vi "RT.vi"   [LabVIEW 2016]
uses:
  rt state control.ctl
  commands.ctl
  <vilib>/FPGAPlugInAG/cRIO-9067/niLvFpga_Open_cRIO-9067.vi
  <vilib>/rvi/interface/common/dynamic/niFpgaDynamicAddResources.vi
  <vilib>/Utility/error.llb/Error Cluster From Error Code.vi
  <vilib>/rvi/errors/niLvFpgaAdjustHostInterfaceError.vi
  <vilib>/rvi/interface/nirviOpenFPGA/nirviOpenFPGA.xnode
  FPGA Bitfiles/NSV-events_FPGATarget_test-FPGA_MCVqyRuBWmI.lvbitx
  FPGA.vi
  <vilib>/rvi/interface/nirviReadWriteControl/nirviReadWriteControl.xnode
  NiFpgaLv.dll
  <vilib>/rvi/interface/Simulation/niFpgaSimulationCallBeginRW.vi
  <vilib>/NI_Real-Time Target Support.lvlib
types:
  T1 = typedef "rt state control.ctl" = enum16{"initialize", "wait for update", "process update", "stop"}
  T2 = typedef "commands.ctl" = enum16{"Flash Both", "Stop All Flash", "Flash FPGA", "Stop FPGA Flash", "Flash RT", "Stop RT Flash"}
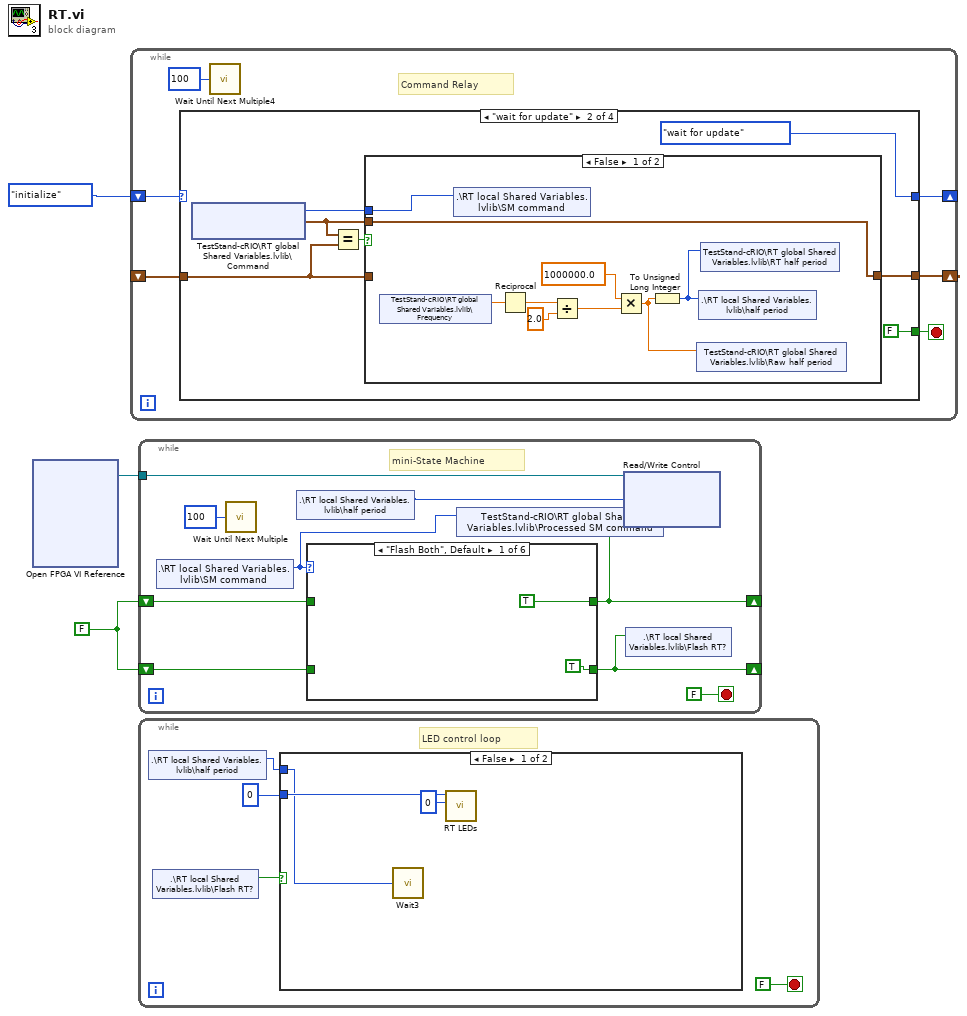
[diagram p0: block diagram]
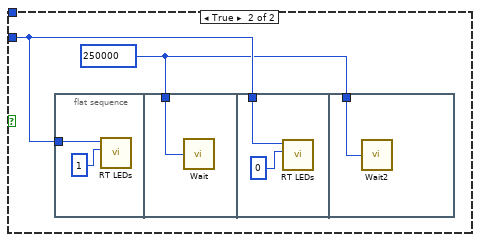
[diagram p2: hidden frame]
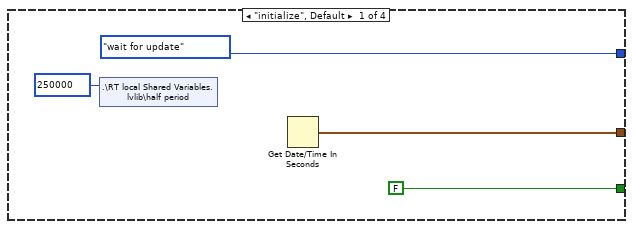
[diagram p3: hidden frame]
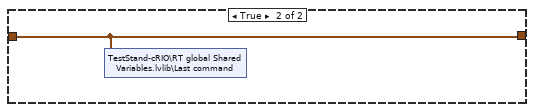
[diagram p4: hidden frame]
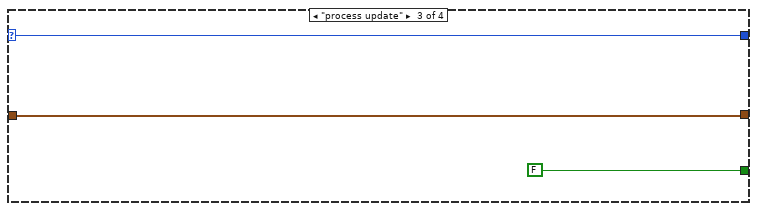
[diagram p5: hidden frame]
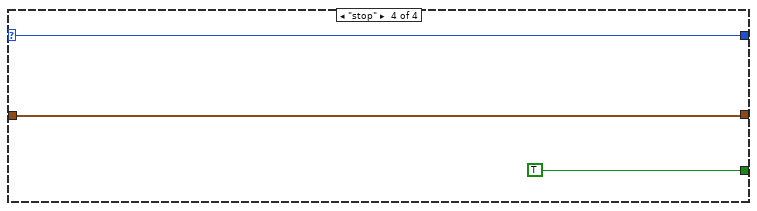
[diagram p6: hidden frame]
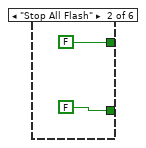
[diagram p7: hidden frame]
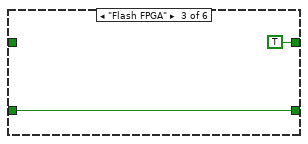
[diagram p8: hidden frame]
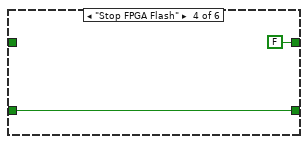
[diagram p9: hidden frame]
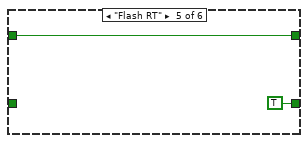
[diagram p10: hidden frame]
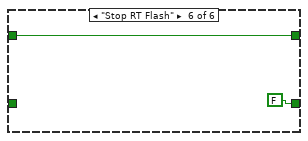
[diagram p11: hidden frame]
diagram:
  w2 = FALSE
  n1 = xnode "Open FPGA VI Reference"() -> ("FPGA VI Reference Out"=w3:refnum<k20>)  [unwired: 2 in, 1 out]
  n2 = while {
    shift-right: [w7] -> _
    shift-left: rt_state_control."initialize" -> [w9]
    shift-right: [w6] -> _
    shift-left: _ -> [w5]
    stop <- w8 stop-if-true
    # "Command Relay"
    n3 = case shown="\"wait for update\"" w9 {
      selector: w9 -> [_ _ w31 w34]
      tunnel: [FALSE FALSE FALSE TRUE] -> w8
      tunnel: [rt_state_control."wait for update" rt_state_control."wait for update" w31 w34] -> w7
      tunnel: [w11 w15 w32 w35] -> w6
      tunnel: w5 -> [_ w16 w32 w35]
      frame "initialize", Default {
        n4 = shared-variable ".\\RT local Shared Variables.lvlib\\half period"(u32 250000 ("half period")) -> ()  [unwired: 1 in, 1 out]
        n5 = Get Date/Time In Seconds() -> (seconds since 1Jan1904=w11:timestamp)
      }
      frame "wait for update" {
        n6 = shared-variable "TestStand-cRIO\\RT global Shared Variables.lvlib\\Command"() -> (w19:T2, w17:timestamp)  [unwired: 1 in, 1 out]
        n7 = Equal?(x=w17, y=w16) -> (x = y?=w18:bool)
        n8 = case shown="False" w18 {
          tunnel: w19 -> [w28 _]
          tunnel: w17 -> [w29 _]
          tunnel: w16 -> [_ w30]
          tunnel: [w29 w30] -> w15
          frame False {
            n9 = shared-variable "TestStand-cRIO\\RT global Shared Variables.lvlib\\Frequency"() -> (w27:dbl)  [unwired: 1 in, 1 out]
            n10 = shared-variable ".\\RT local Shared Variables.lvlib\\SM command"(w28) -> ()  [unwired: 1 in, 1 out]
            n11 = Reciprocal(x=w27) -> (1/x=w26:dbl)
            n12 = Divide(x=w26, y=2.0) -> (x/y=w24:dbl)
            n13 = Multiply(x=1000000.0, y=w24) -> (x*y=w22:dbl)
            n14 = To Unsigned Long Integer(number=w22) -> (unsigned 32bit integer=w21:u32)
            n15 = shared-variable "TestStand-cRIO\\RT global Shared Variables.lvlib\\Raw half period"(w22) -> ()  [unwired: 1 in, 1 out]
            n16 = shared-variable ".\\RT local Shared Variables.lvlib\\half period"(w21) -> ()  [unwired: 1 in, 1 out]
            n17 = shared-variable "TestStand-cRIO\\RT global Shared Variables.lvlib\\RT half period"(w21) -> ()  [unwired: 1 in, 1 out]
          }
          frame True {
            n18 = shared-variable "TestStand-cRIO\\RT global Shared Variables.lvlib\\Last command"(w30) -> ()  [unwired: 1 in, 1 out]
          }
        }
      }
      frame "process update" {
      }
      frame "stop" {
      }
    }
    n19 = call "Wait Until Next Multiple4"("Count(mSec)"=u32 100) -> ()  [unwired: 1 out]
  }
  n20 = while {
    tunnel: w3 -> [w44]
    shift-right: [w43] -> _
    shift-left: w2 -> [w40]
    shift-right: [w42] -> _
    shift-left: w2 -> [w41]
    stop <- FALSE stop-if-true
    # "mini-State Machine"
    n21 = shared-variable ".\\RT local Shared Variables.lvlib\\SM command"() -> (w37:T2)  [unwired: 1 in, 1 out]
    n22 = call "Wait Until Next Multiple"("Count(mSec)"=u32 100) -> ()  [unwired: 1 out]
    n23 = shared-variable ".\\RT local Shared Variables.lvlib\\half period"() -> (w38:u32)  [unwired: 1 in, 1 out]
    n24 = case shown="\"Flash Both\", Default" w37 {
      tunnel: [TRUE ("Boolean") FALSE TRUE FALSE w54 w56] -> w43
      tunnel: [TRUE FALSE w50 w52 TRUE FALSE] -> w42
      tunnel: w41 -> [_ _ w50 w52 _ _]
      tunnel: w40 -> [_ _ _ _ w54 w56]
      frame "Flash Both", Default {
      }
      frame "Stop All Flash" {
      }
      frame "Flash FPGA" {
      }
      frame "Stop FPGA Flash" {
      }
      frame "Flash RT" {
      }
      frame "Stop RT Flash" {
      }
    }
    n25 = shared-variable "TestStand-cRIO\\RT global Shared Variables.lvlib\\Processed SM command"(w37) -> ()  [unwired: 1 in, 1 out]
    n26 = xnode "Read/Write Control"("FPGA VI Reference In"=w44, "Half-period"=w38, "Flash"=w43) -> ()  [unwired: 1 in, 2 out]
    n27 = shared-variable ".\\RT local Shared Variables.lvlib\\Flash RT?"(w42) -> ()  [unwired: 1 in, 1 out]
  }
  n28 = while {
    stop <- FALSE stop-if-true
    # "LED control loop"
    n29 = shared-variable ".\\RT local Shared Variables.lvlib\\half period"() -> (w58:u32)  [unwired: 1 in, 1 out]
    n30 = shared-variable ".\\RT local Shared Variables.lvlib\\Flash RT?"() -> (w60:bool)  [unwired: 1 in, 1 out]
    n31 = case shown="False" w60 {
      tunnel: 0 -> [w64 w66]
      tunnel: w58 -> [w62 _]
      frame False {
        n32 = call "Wait3"("Count(uSec)"=w62) -> ()  [unwired: 1 out]
        n33 = call <vilib>:"RT LEDs.vi"("State"=0, "LED Num"=w64) -> ()  [unwired: 4 in, 2 out]
      }
      frame True {
        w65 = u32 250000 ("UInt32")
        n34 = flat-sequence {
          tunnel: w66 -> [w68]
          tunnel: w65 -> [w69]
          tunnel: w66 -> [w71]
          tunnel: w65 -> [w72]
          frame #0 {
            n35 = call <vilib>:"RT LEDs.vi"("State"=1, "LED Num"=w68) -> ()  [unwired: 4 in, 2 out]
          }
          frame #1 {
            n36 = call "Wait"("Count(uSec)"=w69) -> ()  [unwired: 1 out]
          }
          frame #2 {
            n37 = call <vilib>:"RT LEDs.vi"("State"=0, "LED Num"=w71) -> ()  [unwired: 4 in, 2 out]
          }
          frame #3 {
            n38 = call "Wait2"("Count(uSec)"=w72) -> ()  [unwired: 1 out]
          }
        }
      }
    }
  }
